vi "Add RT to RT Message.vi"(4 "create timestamp channel":bool, 6 "parameters":T2(array[cluster]), 7 "number of words":u16=1, 8 "error in":errorcluster, 9 "remote terminals":cluster{"Rx":T3, "Tx":T3}, 10 "name":string, 11 "port in":T5 format="%.0x") -> (0 "error out":errorcluster, 3 "port out":T5 format="%.0x")   [LabVIEW 2020, in "Ballard MIL-STD-1553 Scripting.lvlib"]
uses:
  <vilib>/NI VeriStand/Custom Device API/Custom Device Item Ref.ctl
  Shared/Terminal Endpoint.ctl
  Shared/Address.ctl
  Shared/Parameter Definition.ctl
  Shared/Direction.ctl
  Ballard MIL-STD-1553 Scripting.lvlib
  <vilib>/NI VeriStand/Custom Device API/Custom Device API.lvlib
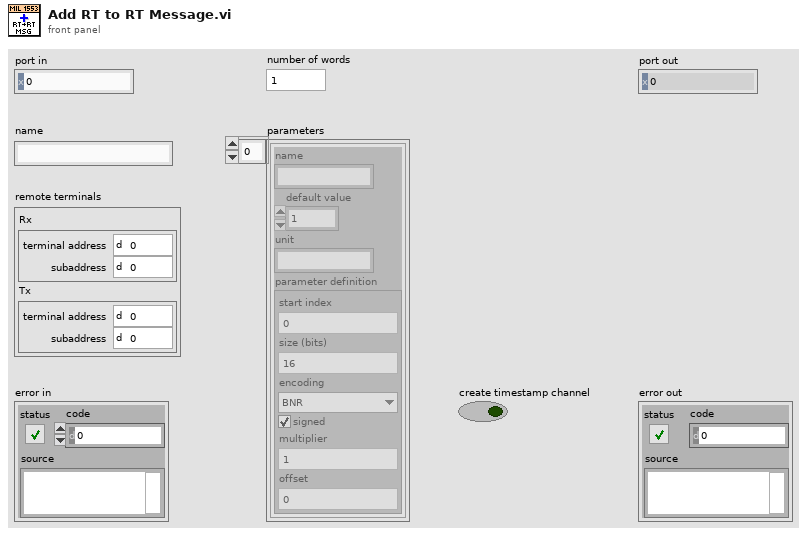
[diagram p1: front panel]
types:
  T1 = typedef "Parameter Definition.ctl" = cluster{"start index":i32, "size (bits)":i32, "encoding":enum16{"BNR", "BCD", "Discrete"}, "signed":bool, "multiplier":dbl, "offset":dbl}
  T2 = cluster{"name":string, "default value":dbl, "unit":string, "parameter definition":T1}[]
  T3 = typedef "Terminal Endpoint.ctl" = cluster{"terminal address":T4, "subaddress":T4}
  T4 = typedef "Address.ctl" = u16
  T5 = typedef "Custom Device API.lvlib/Custom Device Item Ref.ctl" = u64
  T6 = typedef "Direction.ctl" = enum16{"Rx", "Tx"}
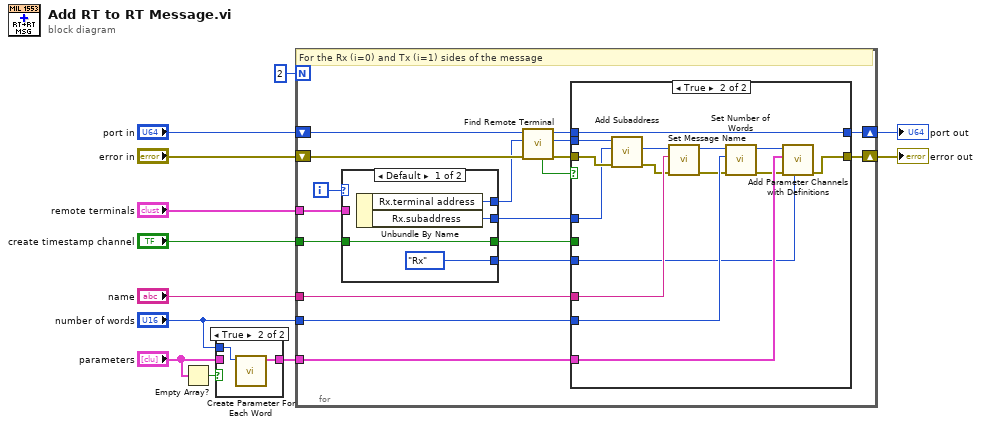
[diagram p0: block diagram]
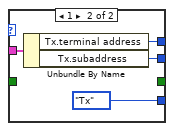
[diagram p2: hidden frame]
diagram:
  n1 = Empty Array?(array="parameters") -> (empty?=w6:bool)
  n2 = case shown="True" w6 {
    tunnel: "number of words" -> [_ w15]
    tunnel: "parameters" -> [w13 _]
    tunnel: [w13 w14] -> w3
    frame False {
    }
    frame True {
      n3 = call "Create Parameter For Each Word.vi"("number of words"=w15) -> ("parameters"=w14:T2)  [unwired: 9 in, 1 out]
    }
  }
  n4 = for {
    N: 2 -> [_]
    tunnel: "create timestamp channel" -> [w17]
    tunnel: "name" -> [w25]
    tunnel: "number of words" -> [w24]
    tunnel: w3 -> [w23]
    shift-right: [w26] -> w8
    shift-left: "port in" -> [w33]
    shift-right: [w27] -> w9
    shift-left: "error in" -> [w32]
    tunnel: "remote terminals" -> [w21]
    i -> [w22]
    # "For the Rx (i=0) and Tx (i=1) sides of the message"
    n5 = case shown="Default" w22 {
      tunnel: w21 -> [_ w41]
      tunnel: [w37 w40] -> w20
      tunnel: [w36 w39] -> w19
      tunnel: [Direction."Rx" Direction."Tx"] -> w18
      tunnel: [w34 _] -> w16
      tunnel: w17 -> [w34 _]
      frame Default {
        n6 = Unbundle By Name() -> ("Rx.terminal address"=w37:T4, "Rx.subaddress"=w36:T4)  [unwired: 1 in]
      }
      frame 1 {
        n7 = Unbundle By Name(w41) -> ("Tx.terminal address"=w40:T4, "Tx.subaddress"=w39:T4)
      }
    }
    n8 = call "Find Remote Terminal.vi"("error in"=w32, "terminal address"=w20, "port in"=w33) -> ("error out"=w28:errorcluster, "remote terminal"=w29:T5, "port out"=w30:T5, "found?"=w31:bool)  [unwired: 5 in]
    n9 = case shown="True" w31 {
      tunnel: w30 -> [w43 w57]
      tunnel: w29 -> [_ w56]
      tunnel: w28 -> [w42 w58]
      tunnel: [w42 w53] -> w27
      tunnel: [w43 w57] -> w26
      tunnel: w19 -> [_ w55]
      tunnel: w24 -> [_ w54]
      tunnel: w23 -> [_ w52]
      tunnel: w25 -> [_ w51]
      tunnel: w18 -> [_ w44]
      tunnel: w16 -> [_ _]
      frame False {
      }
      frame True {
        n10 = call "Add Subaddress.vi"("error in"=w58, "subaddress"=w55, "remote terminal in"=w56) -> ("error out"=w49:errorcluster, "subaddress ref"=w50:T5)  [unwired: 6 in, 1 out]
        n11 = call "Set Message Name.vi"("error in"=w49, "message name"=w51, "message in"=w50) -> ("error out"=w47:errorcluster, "message out"=w48:T5)  [unwired: 7 in]
        n12 = call "Set Number of Words.vi"("error in"=w47, "number of words"=w54, "message in"=w48) -> ("error out"=w45:errorcluster, "message out"=w46:T5)  [unwired: 7 in]
        n13 = call "Add Parameter Channels with Definitions.vi"("direction"=w44, "error in"=w45, "parameters"=w52, "message in"=w46) -> ("error out"=w53:errorcluster)  [unwired: 6 in, 1 out]
      }
    }
  }
  "error out" <- w9
  "port out" <- w8
